vi "Initialize.vi"(8 "error in":errorcluster, 10 "shared resources":refnum<class "Shared Resources.lvclass">, 11 "Execution Unit Implementation in":refnum<class "Execution Unit.lvclass">) -> (0 "error out":errorcluster, 3 "Execution Unit Implementation out":refnum<class "Execution Unit.lvclass">)   [LabVIEW 2020, in "Ballard MIL-STD-1553 Engine.lvlib" / "Implementation.lvlib" / "Execution Unit.lvclass"]
uses:
  Execution Unit.lvclass
  Interfaces/Shared Resources/Shared Resources.lvclass
  Shared Resources/Shared Resources.lvclass
  Shared Resources/Shared Resources.lvclass/Shared Resources.ctl
  Execution Unit.lvclass/Execution Unit.ctl
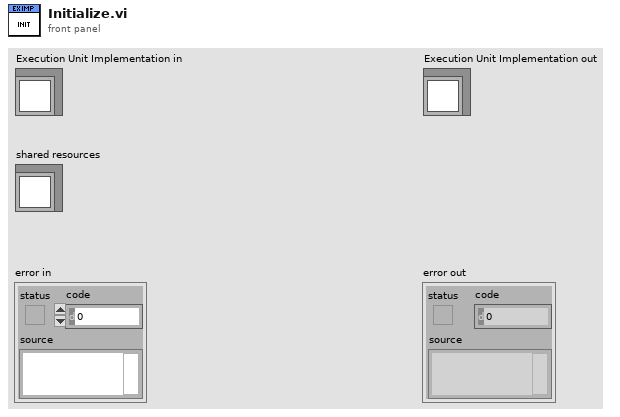
[diagram p1: front panel]
types:
  T1 = typedef "Ballard MIL-STD-1553 Engine.lvlib/Custom Device.lvlib/Hardware Handles.ctl" = cluster{"core handle":u64, "core reader handle":u64, "channel handles":u64[]}
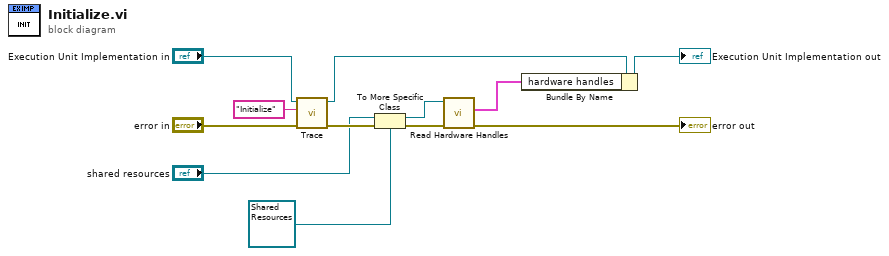
[diagram p0: block diagram]
diagram:
  n1 = call "Trace.vi"("Execution Unit Implementation in"="Execution Unit Implementation in", "message"="Initialize" ("input 2"), "error in (no error)"="error in") -> ("Execution Unit Implementation out"=w3:refnum<class "Execution Unit.lvclass">, "error out"=w8:errorcluster)  [unwired: 6 in]
  n2 = To More Specific Class(target class=refnum<class "Shared Resources.lvclass"> refnum ("Shared Resources in"), reference="shared resources", error in=w8) -> (specific class reference=w4:refnum<class "Shared Resources.lvclass">, error out=w7:errorcluster)
  n3 = call "Read Hardware Handles.vi"("error in"=w7, "Shared Resources in"=w4) -> ("error out"=→"error out":errorcluster, "hardware handles"=w1:T1)  [unwired: 7 in, 1 out]
  n4 = Bundle By Name(cluster=w3, "hardware handles"=w1) -> (→"Execution Unit Implementation out":refnum<class "Execution Unit.lvclass">)
